vi "config_file_check.vi"(8 "error in (no error)":errorcluster, 10 "reference cluster in":T1, 11 "configuration file path":path) -> (0 "error out":errorcluster, 2 "reference cluster out":T1)   [LabVIEW 2016]
uses:
  Type Definitions/reference_cluster.ctl
  Type Definitions/vars_settings.ctl
  Type Definitions/stim_type.ctl
  Type Definitions/backlight_type.ctl
  Type Definitions/vars_runtime.ctl
  Type Definitions/data.ctl
  Type Definitions/notifier_elements_GUI.ctl
  Type Definitions/notifier_elements_DAQ.ctl
  Type Definitions/notifier_elements_write.ctl
  Type Definitions/control_references.ctl
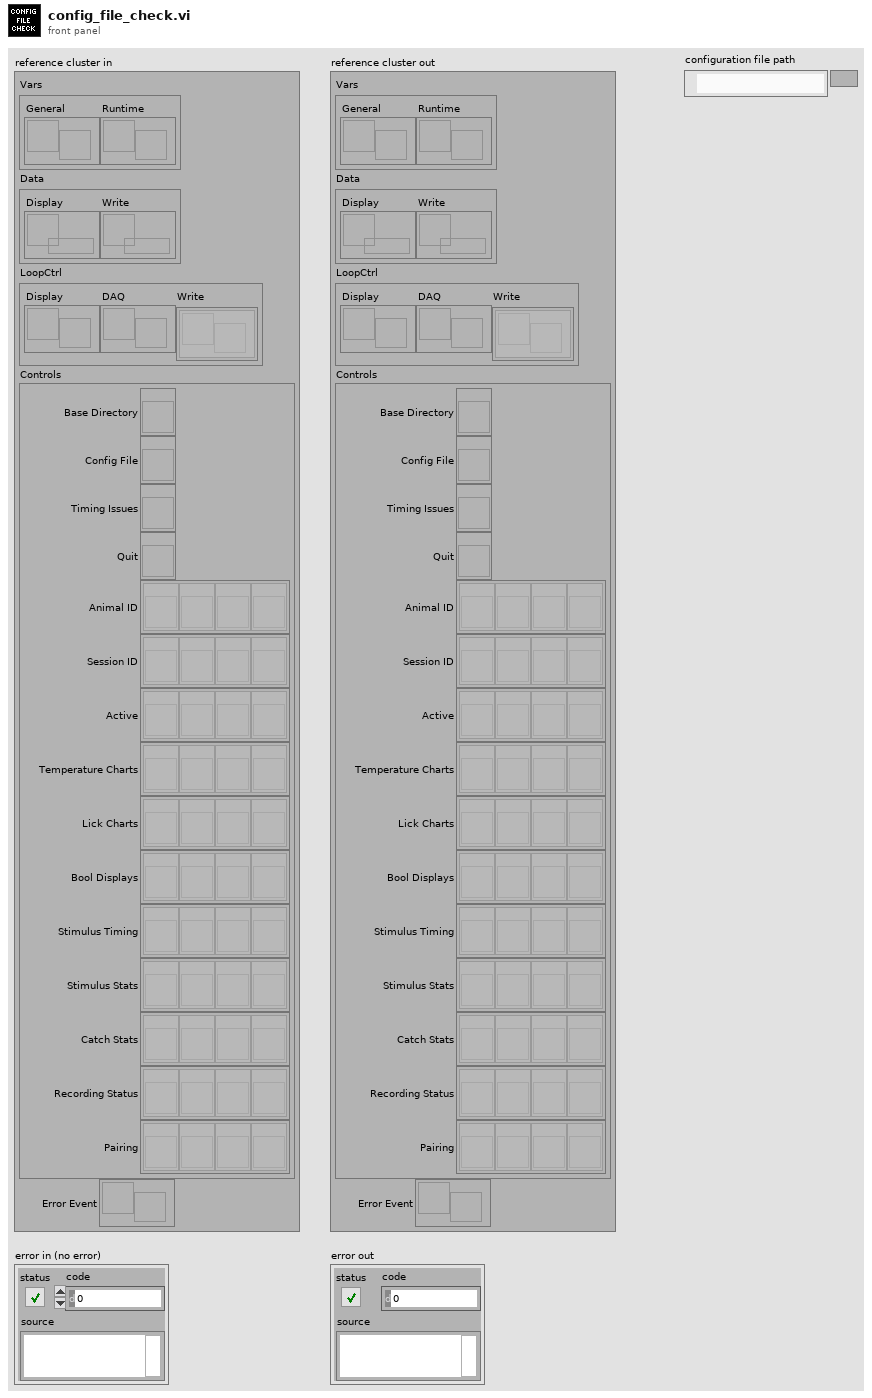
[diagram p1: front panel]
types:
  T1 = typedef "reference_cluster.ctl" = cluster{"Vars":cluster{"General":refnum<notifier>, "Runtime":refnum<notifier>}, "Data":cluster{"Display":refnum<queue>, "Write":refnum<queue>}, "LoopCtrl":cluster{"Display":refnum<notifier>, "DAQ":refnum<notifier>, "Write":refnum<notifier>[]}, "Controls":T2, "Error Event":refnum<user-event>}
  T2 = typedef "control_references.ctl" = cluster{"Base Directory":refnum<vi>, "Config File":refnum<vi>, "Timing Issues":refnum<vi>, "Quit":refnum<vi>, "Animal ID":refnum<vi>[], "Session ID":refnum<vi>[], "Active":refnum<vi>[], "Temperature Charts":refnum<vi>[], "Lick Charts":refnum<vi>[], "Bool Displays":refnum<vi>[], "Stimulus Timing":refnum<vi>[], "Stimulus Stats":refnum<vi>[], "Catch Stats":refnum<vi>[], "Recording Status":refnum<vi>[], "Pairing":refnum<vi>[]}
  T3 = typedef "vars_settings.ctl" = cluster{"base directory":path, "data directory":path, "active":bool, "running":bool, "pairing":bool, "clean tubes":bool, "animal ID":u16, "session ID":u16, "base temp":dbl, "d wait min":u16, "d wait max":u16, "d timeout":u16, "d timeout catch":u16, "d penalty":u16, "d reward":u16, "n reward":u16, "idx stim":u16, "timeout win":u16, "lick win":i32[], "stim type":T4[], "stim dur":u16[], "stim amp":dbl[], "stim freq":u16[], "stim ramp":u16[], "stim catch":u8[], "pairing delay":i16[], "square dur":u16[], "square delay":i16[], "square freq":u8[], "square dc":u8[], "stim shape":dbl[][], "square shape":bool[][], "backlight type":T5, "backlight freq":u16, "dStimOne dur":u16[], "dStimOne delay":i16[], "dStimTwo dur":u16[], "dStimTwo delay":i16[]}
  T4 = typedef "stim_type.ctl" = enum16{"pulse", "vibration", "square", "sine"}
  T5 = typedef "backlight_type.ctl" = enum16{"none", "random", "regular"}
  T6 = cluster{"stim amp":dbl[], "stim dur":u16[], "stim ramp":u16[], "stim freq":u16[], "stim catch":u8[], "square dur":u16[], "square delay":i16[], "square freq":u8[], "square dc":u8[], "dStimOne dur":u16[], "dStimOne delay":i16[], "dStimTwo dur":u16[], "dStimTwo delay":i16[], "pairing delay":i16[]}
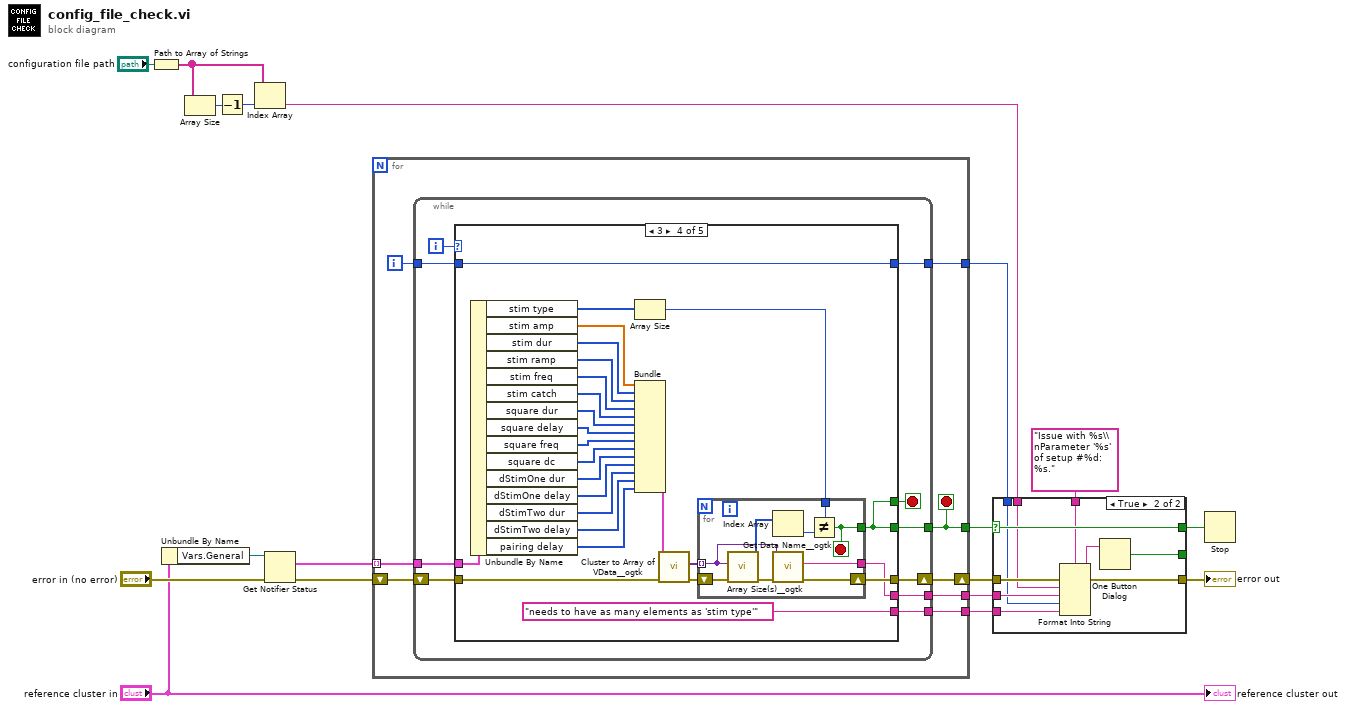
[diagram p0: block diagram]
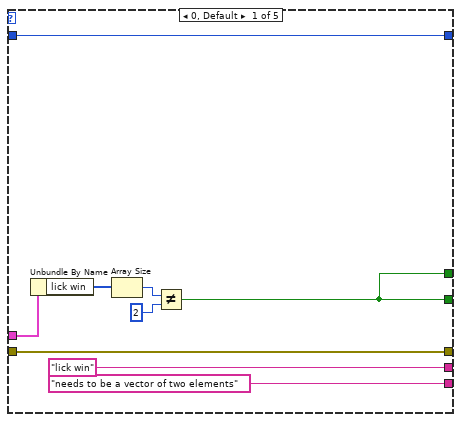
[diagram p3: hidden frame]
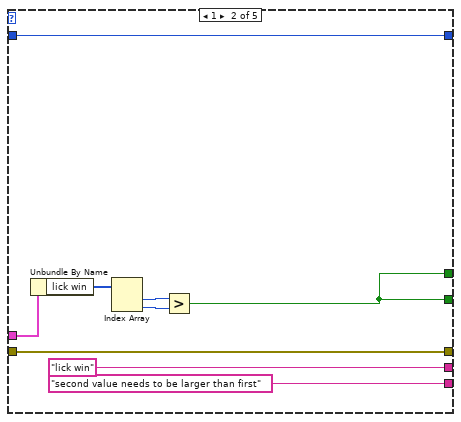
[diagram p4: hidden frame]
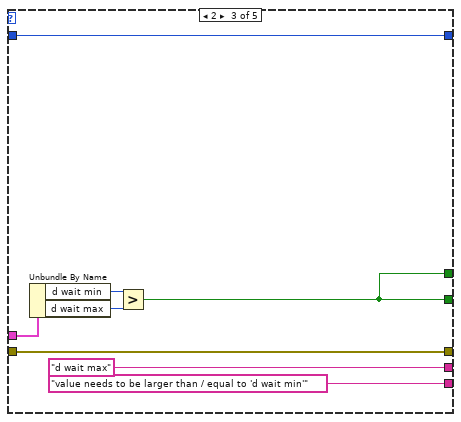
[diagram p5: hidden frame]
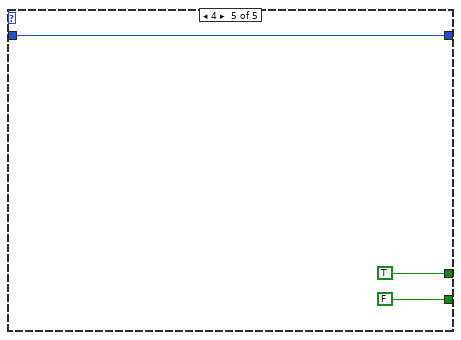
[diagram p6: hidden frame]
diagram:
  n1 = Path to Array of Strings(0:"configuration file path") -> (2:w4:string[])  [unwired: 1 out]
  n2 = Unbundle By Name("reference cluster in") -> ("Vars.General"=w18:refnum<notifier>)
  n3 = Array Size(array=w4) -> (size(s)=w5:i32)
  n4 = Decrement(x=w5) -> (x-1=w6:i32)
  n5 = Index Array(array=w4, index=w6) -> (element=w2:string)
  n6 = Get Notifier Status(notifier=w18, error in (no error)="error in (no error)") -> (current notification=w15:T3[], error out=w16:errorcluster)  [unwired: 3 out]
  n7 = for {
    shift-right: [w25] -> w10
    shift-left: w16 -> [w26]
    tunnel: w15 -> [w24] mode=indexing
    tunnel: [w22] -> w13
    tunnel: [w21] -> w14
    tunnel: [w20] -> w12
    tunnel: [w19] -> w7
    i -> [w23]
    stop <- w21 stop-if-true
    n8 = while {
      shift-right: [w32] -> w25
      shift-left: w26 -> [w33]
      tunnel: w24 -> [w35]
      tunnel: w23 -> [w34]
      tunnel: [w31] -> w22
      tunnel: [w30] -> w21
      tunnel: [w28] -> w20
      tunnel: [w27] -> w19
      i -> [w36]
      stop <- w29 stop-if-true
      n9 = case shown="3" w36 {
        tunnel: w35 -> [w45 w54 w62 w88 _]
        tunnel: [w42 w46 w57 w81 FALSE] -> w30
        tunnel: w34 -> [w41 w53 w61 w87 w98]
        tunnel: w33 -> [w39 w52 w60 w74 _]
        tunnel: [w39 w52 w60 w85 _] -> w32
        tunnel: ["lick win" "lick win" "d wait max" w84 _] -> w31
        tunnel: [w42 w46 w57 w81 TRUE] -> w29
        tunnel: [w41 w53 w61 w87 w98] -> w28
        tunnel: ["needs to be a vector of two elements" "second value needs to be larger than first" "value needs to be larger than / equal to 'd wait min'" "needs to have as many elements as 'stim type'" _] -> w27
        frame 0, Default {
          n10 = Unbundle By Name(w45) -> ("lick win"=w40:i32[])
          n11 = Array Size(array=w40) -> (size(s)=w44:i32)
          n12 = Not Equal?(x=w44, y=2) -> (x != y?=w42:bool)
        }
        frame 1 {
          n13 = Unbundle By Name(w54) -> ("lick win"=w49:i32[])
          n14 = Index Array(array=w49) -> (element #1=w48:i32, element #2=w47:i32)  [unwired: 2 in]
          n15 = Greater?(x=w48, y=w47) -> (0:w46:bool)
        }
        frame 2 {
          n16 = Unbundle By Name(w62) -> ("d wait min"=w56:u16, "d wait max"=w55:u16)
          n17 = Greater?(x=w56, y=w55) -> (0:w57:bool)
        }
        frame 3 {
          n18 = Unbundle By Name(w88) -> ("stim type"=w83:T4[], "stim amp"=w80:dbl[], "stim dur"=w79:u16[], "stim ramp"=w78:u16[], "stim freq"=w77:u16[], "stim catch"=w72:u8[], "square dur"=w71:u16[], "square delay"=w70:i16[], "square freq"=w69:u8[], "square dc"=w68:u8[], "dStimOne dur"=w67:u16[], "dStimOne delay"=w66:i16[], "dStimTwo dur"=w65:u16[], "dStimTwo delay"=w64:i16[], "pairing delay"=w63:i16[])
          n19 = Array Size(array=w83) -> (size(s)=w82:i32)
          n20 = Bundle("stim amp"=w80, "stim dur"=w79, "stim ramp"=w78, "stim freq"=w77, "stim catch"=w72, "square dur"=w71, "square delay"=w70, "square freq"=w69, "square dc"=w68, "dStimOne dur"=w67, "dStimOne delay"=w66, "dStimTwo dur"=w65, "dStimTwo delay"=w64, "pairing delay"=w63) -> (w76:T6)  [unwired: 1 in]
          n21 = call <userlib>:"Cluster to Array of VData__ogtk.vi"("error in (no error)"=w74, "Cluster"=w76) -> ("error out"=w73:errorcluster, "Array of VData"=w75:variant[])  [unwired: 8 in]
          n22 = for {
            shift-right: [w97] -> w85
            shift-left: w73 -> [w90]
            tunnel: [w96] -> w84
            tunnel: w82 -> [w95]
            tunnel: [w94] -> w81
            tunnel: w75 -> [w91] mode=indexing
            stop <- w94 stop-if-true
            n23 = call <userlib>:"Array Size(s)__ogtk.vi"("error in (no error)"=w90, "Array"=w91) -> ("error out"=w89:errorcluster, "Size(s)"=w93:u32[])  [unwired: 7 in, 1 out]
            n24 = Index Array(array=w93) -> (element=w92:u32)  [unwired: 1 in]
            n25 = call <userlib>:"Get Data Name__ogtk.vi"("error in (no error)"=w89, "Data"=w91) -> ("error out"=w97:errorcluster, "Data Name"=w96:string)  [unwired: 7 in, 1 out]
            n26 = Not Equal?(x=w95, y=w92) -> (x != y?=w94:bool)
          }
        }
        frame 4 {
        }
      }
    }
  }
  n27 = case shown="True" w14 {
    selector: w14 -> [w101 w112]
    tunnel: w13 -> [_ w106]
    tunnel: w12 -> [_ w105]
    tunnel: [w101 w112] -> w11
    tunnel: [_ w111] -> _
    tunnel: [w102 w109] -> w9
    tunnel: w10 -> [w102 w110]
    tunnel: w7 -> [_ w107]
    tunnel: w2 -> [_ w104]
    tunnel: "Issue with %s\\nParameter '%s' of setup #%d: %s." -> [_ w103]
    frame False {
    }
    frame True {
      n28 = Format Into String(format string=w103, error in=w110, w104, w106, w105, w107) -> (resulting string=w108:string, error out=w109:errorcluster)  [unwired: 1 in]
      n29 = One Button Dialog(message=w108) -> (true=w111:bool)  [unwired: 1 in]
    }
  }
  "error out" <- w9
  n30 = Stop(stop? (T)=w11) -> ()
  "reference cluster out" <- "reference cluster in"
